vi "Close Group.vi"(10 "group_id":i32, 11 "error in (no error)":errorcluster) -> (3 "error out":errorcluster)   [LabVIEW 2010]
uses:
  Release/HDF5Tools.dll
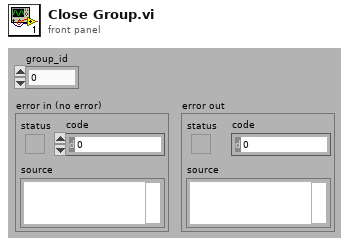
[diagram p1: front panel]
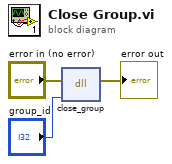
[diagram p0: block diagram]
diagram:
  n1 = dll-call lib="Z:/users/alex/projects/HDF5Tools/Release/HDF5Tools.dll" fn="close_group"(error in="error in (no error)", "group_id"="group_id") -> (error out=→"error out":errorcluster)  [unwired: 4 in, 1 out]
